vi "ReadWrite.Data.Reset.vi"(8 "error in (no error)":errorcluster, 10 "timeout ms":i32, 11 "Ref":T1) -> (0 "error out":errorcluster, 1 "Timeout?":bool)   [LabVIEW 2023, in "Data Access Engine.lvlib" / "Data Access Engine.lvclass"]
uses:
  Data Access Engine.lvclass
  Access Type Classes/ReadWrite/ReadWrite.lvclass
  Access Type Classes/ReadWrite/ReadWrite.lvclass/ReadWrite.ctl
  Types/ReadWrite.DVR.ctl
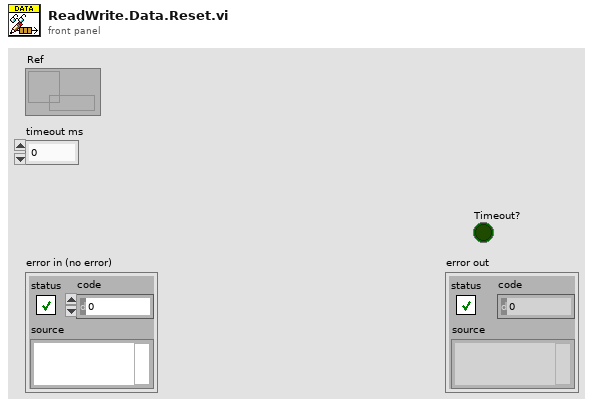
[diagram p1: front panel]
types:
  T1 = typedef "Data Access Engine.lvlib/Data Access Engine.lvclass/ReadWrite.DVR.ctl" = refnum<data-value>
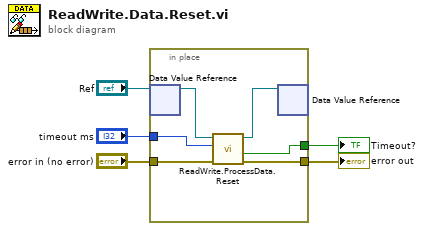
[diagram p0: block diagram]
diagram:
  n1 = in-place {
    in-place-border: "error in (no error)" -> [w9]
    in-place-border: [w6] -> w4
    in-place-border: "timeout ms" -> [w8]
    in-place-border: [w7] -> w1
    n2 = in-place-dvr #1("Ref") -> (w11:refnum<class "ReadWrite.lvclass">)  [unwired: 1 out]
    n3 = call "ReadWrite.ProcessData.Reset.vi"("error in (no error)"=w9, "timeout ms"=w8, "ReadWrite in"=w11) -> ("error out"=w6:errorcluster, "Timeout?"=w7:bool, "ReadWrite out"=w10:refnum<class "ReadWrite.lvclass">)  [unwired: 6 in]
    n4 = in-place-dvr #1(w10) -> ()  [unwired: 2 out]
  }
  "error out" <- w4
  "Timeout?" <- w1
